vi "Test angle.vi"() -> ()   [LabVIEW 2011]
uses:
  <vilib>/express/express arith-compare/Formula/XNode/ExpressFormulaBlockNode.xnode
panel:
  out "Waveform Chart":dbl(graph)
  in  "stop":bool
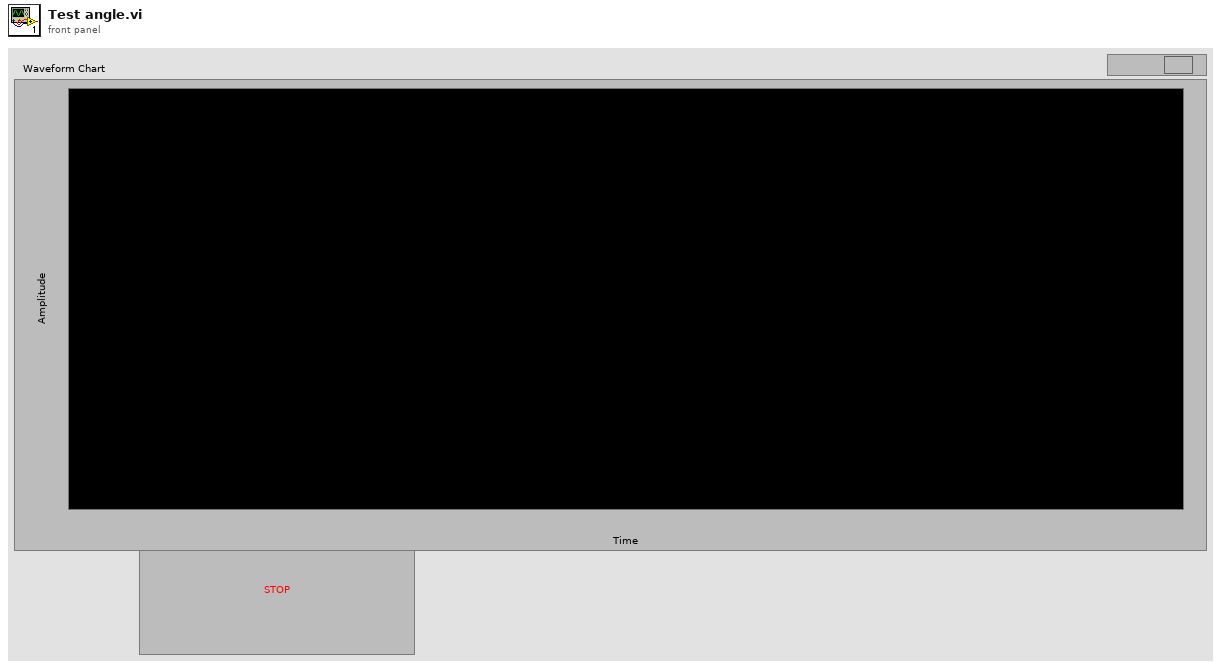
[diagram p1: front panel]
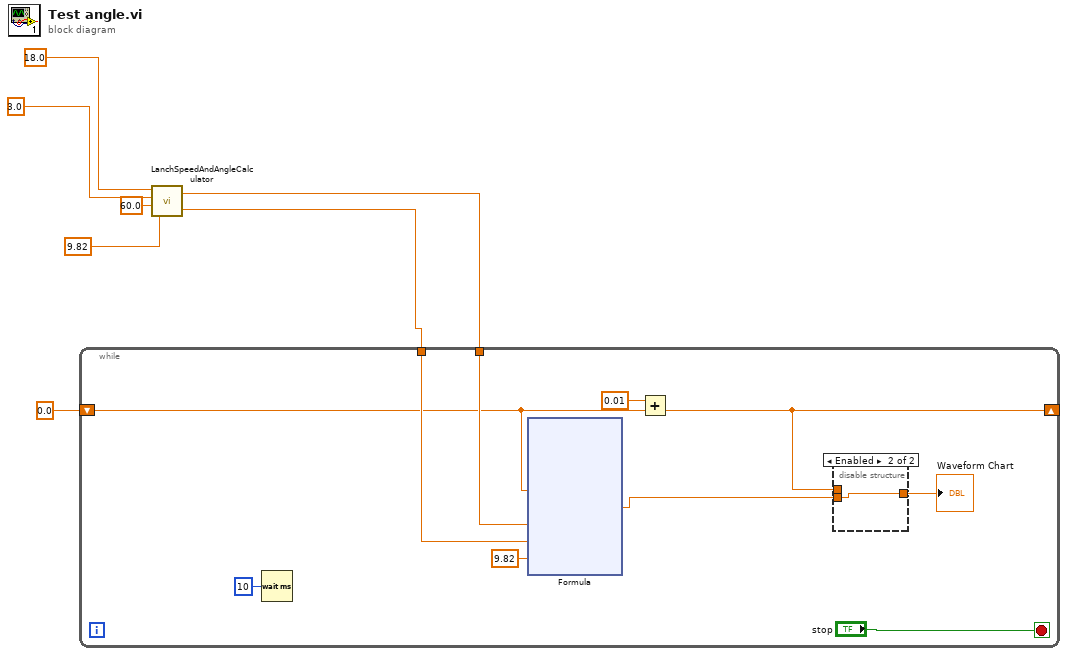
[diagram p0: block diagram]
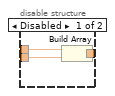
[diagram p2: hidden frame]
diagram:
  n1 = call "LanchSpeedAndAngleCalculator.vi"("g"=9.82, "b"=60.0, "h"=3.0, "d"=18.0) -> ("V"=w1:dbl, "a"=w2:dbl)
  n2 = while {
    tunnel: w1 -> [w16]
    tunnel: w2 -> [w15]
    shift-right: [w9] -> _
    shift-left: 0.0 ("X") -> [w12]
    stop <- "stop" stop-if-true
    n3 = Wait (ms)(milliseconds to wait=u32 10) -> ()  [unwired: 1 out]
    n4 = xnode "Formula"("x"=w12, "a"=w15, "v"=w16, "g"=9.82) -> ("Result"=w8:dbl)  [unwired: 1 in, 1 out]
    n5 = Add(x=0.01, y=w12) -> (x+y=w9:dbl)
    n6 = disable-structure shown="Enabled" {
      disable-tunnel: [w20 w21] -> w10
      disable-tunnel: w9 -> [w19 _]
      disable-tunnel: w8 -> [w18 w21]
      frame Disabled {
        n7 = Build Array(w19, w18) -> (w20:dbl[])
      }
      frame Enabled {
      }
    }
    "Waveform Chart" <- w10
  }
